vi "Parse Sweep Core.vi"(0 "Vector Path Group in":refnum<class "Vector Path Group.lvclass">, 1 "Sweep Name":string, 5 "Config Rows":string[](array[string]), 7 "Power":dbl format="%#_13g", 9 "Frequencies":dbl[](array[numeric]), 11 "error in (no error)":errorcluster) -> (4 "Vector Path Group out":refnum<class "Vector Path Group.lvclass">, 15 "error out":errorcluster)   [LabVIEW 2023, in "RFFixtureCharact.Public.lvlib" / "Vector Path Group.lvclass"]
uses:
  Vector Path Group.lvclass
  Type Definitions/Sweep.ctl
  Common/RFCalAndFixtureCharact.Common.lvlib
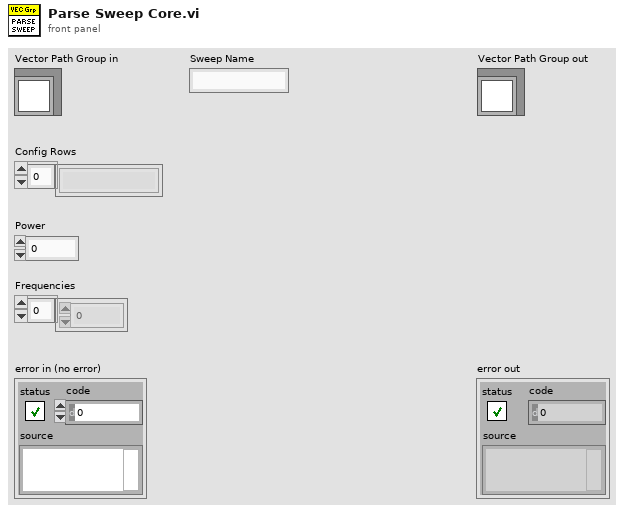
[diagram p1: front panel]
types:
  T1 = typedef "RFFixtureCharact.Public.lvlib/Vector Path Group.lvclass/Sweep.ctl" = cluster{"Port Power":dbl, "Frequencies":dbl[], "Test Receiver Attenuation":dbl, "IF Bandwidth":dbl}
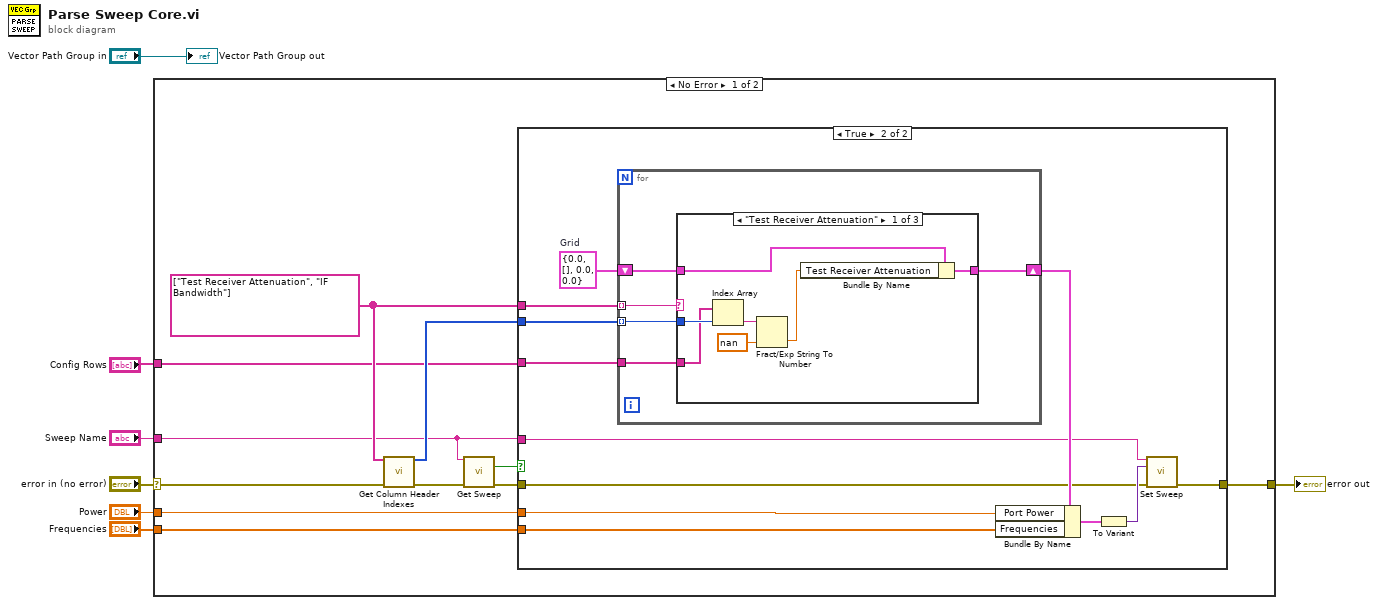
[diagram p0: block diagram]
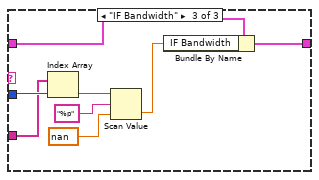
[diagram p4: hidden frame]
diagram:
  n1 = case shown="No Error" "error in (no error)" {
    selector: "error in (no error)" -> [w17 w53]
    tunnel: [w18 w53] -> w5
    tunnel: "Config Rows" -> [w12 _]
    tunnel: "Power" -> [w11 _]
    tunnel: "Frequencies" -> [w10 _]
    tunnel: "Sweep Name" -> [w8 _]
    frame No Error {
      w14 = string[] ["Test Receiver Attenuation", "IF Bandwidth"] ("Column Header Names")
      n2 = call "Get Column Header Indexes.vi"("Column Header Names"=w14, "error in"=w17) -> ("Column Header Indices"=w13:i32[], "error out"=w9:errorcluster)  [unwired: 11 in, 1 out]
      n3 = call "Get Sweep.vi"("Sweep Name"=w8, "error in (no error)"=w9) -> ("Sweep not found?"=w15:bool, "error out"=w16:errorcluster)  [unwired: 11 in, 1 out]
      n4 = case shown="True" w15 {
        tunnel: [w19 w31] -> w18
        tunnel: w16 -> [w19 w22]
        tunnel: w14 -> [_ w30]
        tunnel: w13 -> [_ w28]
        tunnel: w8 -> [_ w26]
        tunnel: w12 -> [_ w23]
        tunnel: w11 -> [_ w21]
        tunnel: w10 -> [_ w20]
        frame False {
        }
        frame True {
          w29 = T1 {"Port Power"=0.0, "Frequencies"=[], "Test Receiver Attenuation"=0.0, "IF Bandwidth"=0.0}  # Grid
          n5 = for {
            tunnel: w30 -> [w36] mode=indexing
            shift-right: [w33] -> w27
            shift-left: w29 -> [w35]
            tunnel: w28 -> [w34] mode=indexing
            tunnel: w23 -> [w32]
            n6 = case shown="\"Test Receiver Attenuation\"" w36 {
              tunnel: w35 -> [w43 w44 w52]
              tunnel: w34 -> [w40 _ w49]
              tunnel: [w42 w44 w51] -> w33
              tunnel: w32 -> [w39 _ w48]
              frame "Test Receiver Attenuation" {
                n7 = Index Array(array=w39, index=w40) -> (element=w38:string)
                n8 = Fract/Exp String To Number(string=w38, default (0 dbl)=nan) -> (number=w41:dbl)  [unwired: 2 in, 1 out]
                n9 = Bundle By Name(cluster=w43, "Test Receiver Attenuation"=w41) -> (w42:T1)
              }
              frame Default {
              }
              frame "IF Bandwidth" {
                n10 = Index Array(array=w48, index=w49) -> (element=w47:string)
                n11 = Scan Value(string=w47, format string="%p", default (0 dbl)=nan) -> (value=w50:dbl)  [unwired: 1 out]
                n12 = Bundle By Name(cluster=w52, "IF Bandwidth"=w50) -> (w51:T1)
              }
            }
          }
          n13 = Bundle By Name(cluster=w27, "Port Power"=w21, "Frequencies"=w20) -> (w24:T1)
          n14 = To Variant(anything=w24) -> (Variant=w25:variant)
          n15 = call "Set Sweep.vi"("Sweep Name"=w26, "Sweep in"=w25, "error in (no error)"=w22) -> ("error out"=w31:errorcluster)  [unwired: 12 in]
        }
      }
    }
    frame Error {
    }
  }
  "error out" <- w5
  "Vector Path Group out" <- "Vector Path Group in"
